vi "Create Plugin Groups.vi"(8 "error in (no error)":errorcluster, 10 "parent tag":string, 11 "Application Data In":T1 {"current buffer data"."channels"."configuration"."string offset" format="%d bytes"; "current buffer data"."avg bandwidth" format="%.0g bytes"}) -> (0 "error out":errorcluster, 1 "async plugins tag":string, 2 "inline plugins tag":string, 3 "Application Data out":T1 {"current buffer data"."channels"."configuration"."string offset" format="%d bytes"; "current buffer data"."avg bandwidth" format="%.0g bytes"})   [LabVIEW 2017, in "Data Viewer.lvlib"]
uses:
  Core/VIs/Data Viewer/Source/Data Viewer.lvlib
  Main VI/Application Data.ctl
  <vilib>/NI/Memory Manager/Classes/Pointer/Pointer.lvclass
  VeriStand/Data Sharing Custom Device/Source/DSF Core.lvlibp/Classes/Configuration/Core/Framework/Framework Configuration.lvclass
  Buffer Reader/Queue Data.ctl
  Buffer Reader/Buffer Data.ctl
  VeriStand/Data Sharing Custom Device/Source/DSF Core.lvlibp/Classes/Configuration/Core/Transfer/Channel Configuration.ctl
  VeriStand/Data Sharing Custom Device/Source/DSF Core.lvlibp/Typedefs/Core Channel Configuration.ctl
  VeriStand/Data Sharing Custom Device/Source/DSF Core.lvlibp/Typedefs/DSF Data Type.ctl
  VeriStand/Data Sharing Custom Device/Source/DSF Core.lvlibp/Typedefs/DSF Settings Info.ctl
  VeriStand/Data Sharing Custom Device/Source/DSF Core.lvlibp/Typedefs/DSF Byte Order.ctl
  VeriStand/Data Sharing Custom Device/Source/DSF Core.lvlibp/Classes/Thread/Data Server/DSF Buffer Subset Descriptor.ctl
  VeriStand/Data Sharing Custom Device/Source/DSF Core.lvlibp/Typedefs/DSF Buffer Type.ctl
  Main VI/Values Channels.ctl
  Tree Item Type.ctl
  VeriStand/Data Sharing Custom Device/Source/DSF Core.lvlibp
  VeriStand/Data Sharing Custom Device/Source/DSF Core.lvlibp/Classes/Configuration/Core/Channel/Channel Configuration.lvclass
  VeriStand/Data Sharing Custom Device/Source/DSF Core.lvlibp/Classes/Configuration/Core/Transfer/Transfer Configuration.lvclass
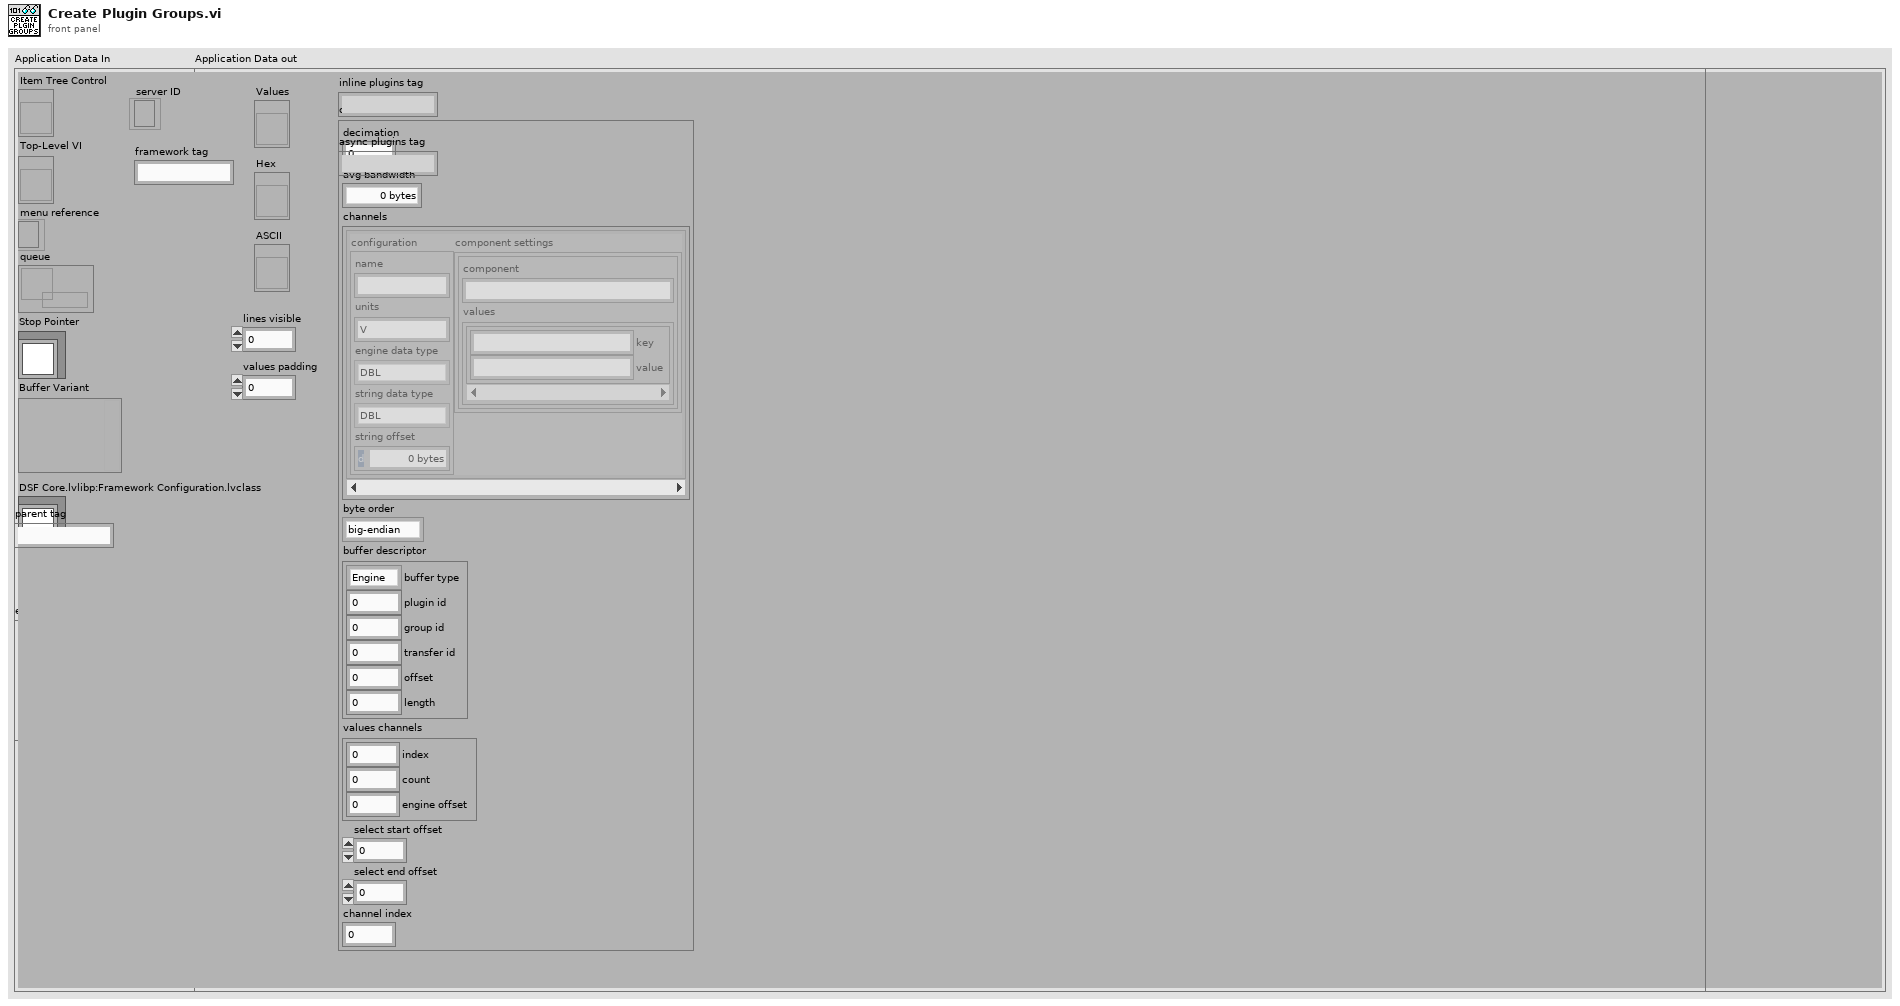
[diagram p1: front panel]
types:
  T1 = typedef "Data Viewer.lvlib/Application Data.ctl" = cluster{"Item Tree Control":refnum<vi>, "Top-Level VI":refnum<vi>, "menu reference":refnum<k9>, "queue":refnum<queue>, "Stop Pointer":refnum<class "Pointer.lvclass">, "Buffer Variant":variant, "server ID":refnum<k5>, "framework tag":string, "Values":refnum<vi>, "Hex":refnum<vi>, "ASCII":refnum<vi>, "lines visible":i32, "values padding":i32, "current buffer data":T2, "DSF Core.lvlibp:Framework Configuration.lvclass":refnum<class "Framework Configuration.lvclass">}
  T2 = typedef "Data Viewer.lvlib/Buffer Data.ctl" = cluster{"decimation":u64, "avg bandwidth":dbl, "channels":T3[], "byte order":T7, "buffer descriptor":T8, "values channels":T10, "select start offset":u64, "select end offset":u64, "channel index":i32}
  T3 = typedef "DSF Core.lvlibp/Transfer Configuration.lvclass/Channel Configuration.ctl" = cluster{"configuration":T4, "component settings":T6[]}
  T4 = typedef "DSF Core.lvlibp/Channel Configuration.lvclass/Core Channel Configuration.ctl" = cluster{"name":string, "units":string, "engine data type":T5, "string data type":T5, "string offset":u64}
  T5 = typedef "DSF Core.lvlibp/DSF Data Type.ctl" = enum8{"Bool", "SGL", "DBL", "I8", "I16", "I32", "I64", "U8", "U16", "U32", "U64"}
  T6 = typedef "DSF Core.lvlibp/DSF Settings Info.ctl" = cluster{"component":string, "values":cluster{"key":string, "value":string}[]}
  T7 = typedef "DSF Core.lvlibp/DSF Byte Order.ctl" = enum8{"big-endian", "little-endian"}
  T8 = typedef "DSF Core.lvlibp/DSF Buffer Subset Descriptor.ctl" = cluster{"buffer type":T9, "plugin id":i32, "group id":i32, "transfer id":i32, "offset":u64, "length":i64}
  T9 = typedef "DSF Core.lvlibp/DSF Buffer Type.ctl" = enum16{"Engine", "String"}
  T10 = typedef "Data Viewer.lvlib/Values Channels.ctl" = cluster{"index":i32, "count":i32, "engine offset":u64}
  T11 = typedef "Data Viewer.lvlib/Tree Item Type.ctl" = enum16{"Framework", "Plugin Group", "Plugin", "Group", "Transfer", "Buffer", "Channel"}
  T12 = typedef "Data Viewer.lvlib/Tree Item.ctl" = cluster{"Left Cell String":string, "Child Text":string[], "Child Tag":string, "Glyph Index":i32}
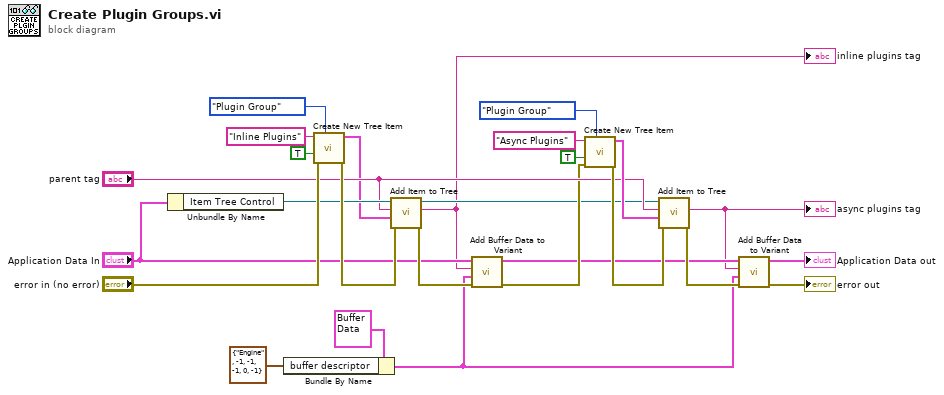
[diagram p0: block diagram]
diagram:
  n1 = Unbundle By Name("Application Data In") -> ("Item Tree Control"=w16:refnum<vi>)
  n2 = Bundle By Name(cluster=T2 {"decimation"=0, "avg bandwidth"=0.0, "channels"=[], "byte order"=enum."big-endian", "buffer descriptor"={"buffer type"=enum."Engine", "plugin id"=0, "group id"=0, "transfer id"=0, "offset"=0, "length"=0}, "values channels"={"index"=0, "count"=0, "engine offset"=0}, "select start offset"=18446744073709551615, "select end offset"=0, "channel index"=-1} ("Buffer data"), "buffer descriptor"=T8 {"buffer type"=enum."Engine", "plugin id"=-1, "group id"=-1, "transfer id"=-1, "offset"=0, "length"=-1}) -> (w2:T2)
  n3 = call "Create New Tree Item.vi"("Item Type"=Tree_Item_Type."Plugin Group", "error in"="error in (no error)", "found?"=TRUE, "Left Cell String"="Inline Plugins") -> ("error out"=w23:errorcluster, "Item"=w14:T12)  [unwired: 6 in]
  n4 = call "Add Item to Tree.vi"("error in (no error)"=w23, "Item"=w14, "parent tag"="parent tag", "TreeControl in"=w16) -> ("error out"=w12:errorcluster, "new item tag"=w9:string, "TreeControl out"=w10:refnum<vi>)  [unwired: 5 in]
  "inline plugins tag" <- w9
  n5 = call "Add Buffer Data to Variant.vi"("error in (no error)"=w12, "Buffer data"=w2, "tag"=w9, "Application Data In in"="Application Data In") -> ("error out"=w13:errorcluster, "Application Data In out"=w5:T1)  [unwired: 6 in]
  n6 = call "Create New Tree Item.vi"("Item Type"=Tree_Item_Type."Plugin Group", "error in"=w13, "found?"=TRUE, "Left Cell String"="Async Plugins") -> ("error out"=w19:errorcluster, "Item"=w18:T12)  [unwired: 6 in]
  n7 = call "Add Item to Tree.vi"("error in (no error)"=w19, "Item"=w18, "parent tag"="parent tag", "TreeControl in"=w10) -> ("error out"=w6:errorcluster, "new item tag"=w4:string)  [unwired: 5 in, 1 out]
  "async plugins tag" <- w4
  n8 = call "Add Buffer Data to Variant.vi"("error in (no error)"=w6, "Buffer data"=w2, "tag"=w4, "Application Data In in"=w5) -> ("error out"=→"error out":errorcluster, "Application Data In out"=→"Application Data out":T1)  [unwired: 6 in]
